vi "Circurit_Switch.vi"(1 "error in (no error)":errorcluster, 2 "Data in":string) -> (0 "error out (no error)":errorcluster)   [LabVIEW 2011]
doc: "This VI switches one component on/off (connect/disconnect)\n\nData in:\n <card><component>\n\nExample: Toggle component 5 on card 2 --> following string 2 5"
uses:
  Server_Globals.vi
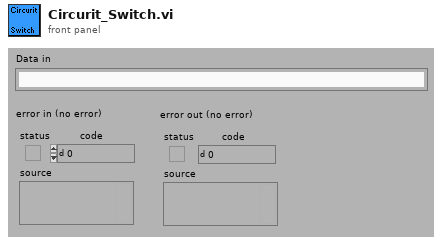
[diagram p1: front panel]
types:
  T1 = cluster{"I/O Settings":u64[], "Instrument Handle":cluster{"5402":refnum<k15>, " 5112":refnum<k15>, "4072":refnum<k15>, "USB":refnum<visa-resource-name>, "4110":refnum<k15>}, "Logfile":refnum<file>, "Log Level":i8, "Clear":i32[], "OS Set":cluster{"instrument handle out":refnum<k15>, "remaining string":string, "Settings":cluster{"Horizontal Conf.":cluster{"Min. Sample rate":dbl, "Reference position":dbl, "Record Length":i16}, "Channel A":cluster{"Enable":bool, "Vertical coupling":dbl, "Vertical range":dbl, "Vertical offset":dbl, "Probe attenuation":dbl}, "Channel B":cluster{"Enable":bool, "Vertical coupling":dbl, "Vertical range":dbl, "Vertical offset":dbl, "Probe attenuation":dbl}, "Trigger":cluster{"Source":enum8{"channel 1", "channel 2", "Imediate", "External trigger"}, "Slope":enum8{"Positive", "Negative"}, "Coupling":enum8{"AC", "DC"}, "Level":dbl, "Holdoff":dbl, "Delay":dbl, " Timeout":dbl, " Mode":enum8{"Normal", "Auto", "Auto Level"}}, "Measurements":cluster{"Measurement 1, Channel":enum8{"Channel 1", "Channel 2", "Channel 3", "Channel 4"}, "Measurement 1, Selection":u16, "Measurement 2, Channel":enum8{"Channel 1", "Channel 2", "Channel 3", "Channel 4"}, "Measurement 2,  Selection":u16, "Measurement 3, Channel":enum8{"Channel 1", "Channel 2", "Channel 3", "Channel 4"}, "Measurement 3, Selection 3":u16}}}, "DC Power Supply":cluster{"0":refnum<k15>, "1":refnum<k15>, "2":refnum<k15>, "3":refnum<k15>, "4":refnum<k15>}, "USB Interface":cluster{"0":refnum<visa-resource-name>, "1":refnum<visa-resource-name>, "2":refnum<visa-resource-name>, "3":refnum<visa-resource-name>, "4":refnum<visa-resource-name>}, "Function Generator":cluster{"0":refnum<k15>, "1":refnum<k15>, "2":refnum<k15>, "3":refnum<k15>, "4":refnum<k15>}, "Digital Multimeter":cluster{"0":refnum<k15>, "1":refnum<k15>, "2":refnum<k15>, "3":refnum<k15>, "4":refnum<k15>}, "Digital Osciliscope":cluster{"0":refnum<k15>, "1":refnum<k15>, "2":refnum<k15>, "3":refnum<k15>, "4":refnum<k15>}, "To M Server":string, "Adres":string[][], "Matrix version":string, "MD5":string, "Digital Multimeter Card 2":cluster{"0":string, "1":string, "2":string, "3":string, "4":string}}
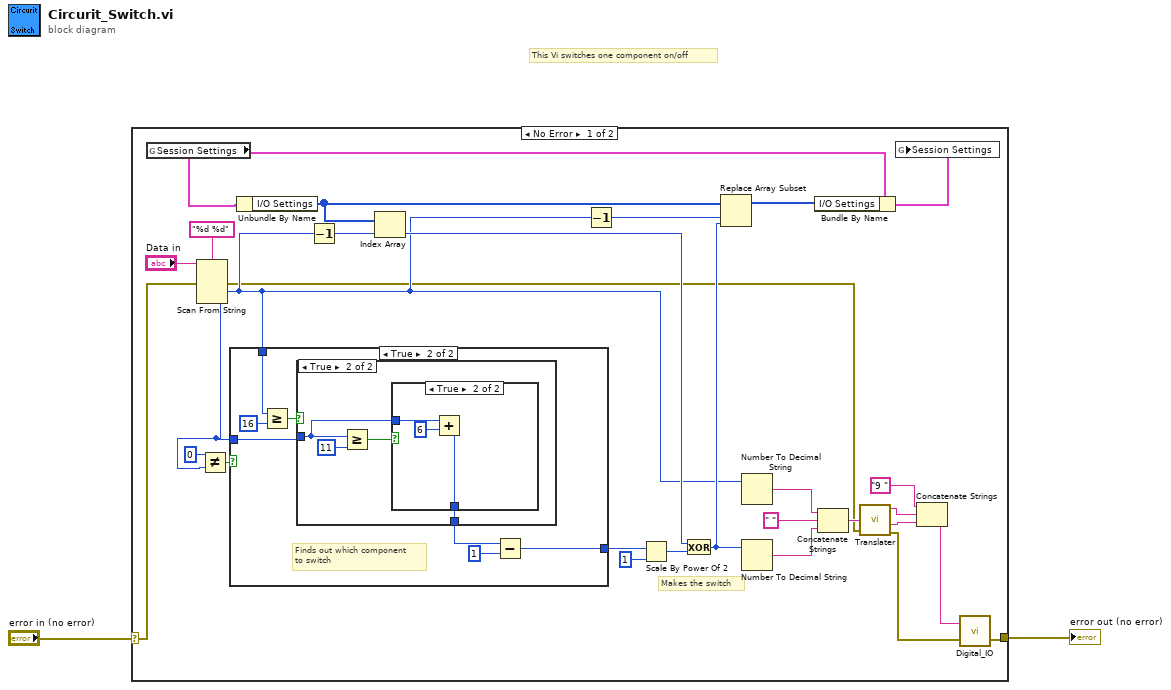
[diagram p0: block diagram]
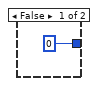
[diagram p2: hidden frame]
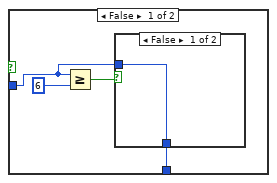
[diagram p3: hidden frame]
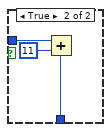
[diagram p4: hidden frame]
diagram:
  # "This Vi switches one component on/off"
  n1 = case shown="No Error" "error in (no error)" {
    selector: "error in (no error)" -> [w5 w56]
    tunnel: [w23 w56] -> w2
    frame No Error {
      # "Makes the switch"
      n2 = global read "Server_Globals.vi" "Session Settings"() -> (w26:T1)
      n3 = Scan From String(format string="%d %d", input string="Data in", error in=w5) -> (error out=w4:errorcluster, output 1=w6:i32, output 2=w20:i32)  [unwired: 3 in, 2 out]
      n4 = Not Equal?(x=0, y=w20) -> (x != y?=w24:bool)
      n5 = case shown="True" w24 {
        tunnel: w20 -> [_ w36]
        tunnel: w6 -> [_ w38]
        tunnel: [0 w33] -> w10
        frame False {
        }
        frame True {
          # "Finds out which component\nto switch"
          n6 = Greater Or Equal?(x=w38, y=16) -> (x >= y?=w37:bool)
          n7 = case shown="True" w37 {
            tunnel: w36 -> [w41 w49]
            tunnel: [w40 w48] -> w35
            frame False {
              n8 = Greater Or Equal?(x=w41, y=6) -> (x >= y?=w43:bool)
              n9 = case shown="False" w43 {
                tunnel: w41 -> [w44 w47]
                tunnel: [w44 w45] -> w40
                frame False {
                }
                frame True {
                  n10 = Add(x=w47, y=11) -> (x+y=w45:i32)
                }
              }
            }
            frame True {
              n11 = Greater Or Equal?(x=w49, y=11) -> (x >= y?=w50:bool)
              n12 = case shown="True" w50 {
                tunnel: w49 -> [w52 w55]
                tunnel: [w52 w53] -> w48
                frame False {
                }
                frame True {
                  n13 = Add(x=w55, y=6) -> (x+y=w53:i32)
                }
              }
            }
          }
          n14 = Subtract(x=w35, y=1) -> (x-y=w33:i32)
        }
      }
      n15 = Unbundle By Name(w26) -> ("I/O Settings"=w29:u64[])
      n16 = Decrement(x=w6) -> (x-1=w8:i32)
      n17 = Index Array(array=w29, index=w8) -> (element=w22:u64)
      n18 = Decrement(x=w6) -> (x-1=w7:i32)
      n19 = Scale By Power Of 2(n=w10, x=1) -> (x*2^n=w11:i32)
      n20 = Exclusive Or(1:w11, 2:w22) -> (0:w18:u64)
      n21 = Replace Array Subset(array=w29, new element=w18, index=w7) -> (w28:u64[])
      n22 = Number To Decimal String(number=w6) -> (decimal integer string=w14:string)  [unwired: 1 in]
      n23 = Number To Decimal String(number=w18) -> (decimal integer string=w13:string)  [unwired: 1 in]
      n24 = Bundle By Name(cluster=w26, "I/O Settings"=w28) -> (w27:T1)
      n25 = Concatenate Strings(w14, " ", w13) -> (w15:string)
      n26 = call "Translater.vi"("In"=w15, "error in (no error)"=w4) -> ("Card"=w17:string, "Comp"=w16:string, "error out (no error)"=w3:errorcluster)  [unwired: 2 in]
      n27 = global write "Server_Globals.vi" "Session Settings"(w27) -> ()
      n28 = Concatenate Strings("9 ", w17, w16) -> (w21:string)
      n29 = call "Digital_IO.vi"("error in"=w3, "Data in"=w21) -> ("error out (no error)"=w23:errorcluster)  [unwired: 1 in]
    }
    frame Error {
    }
  }
  "error out (no error)" <- w2
